vi "Make laser cluster.vi"(0 "445 laser":refnum<visa-resource-name>, 5 "488 laser":refnum<visa-resource-name>, 7 "561 laser":refnum<visa-resource-name>, 9 "640 laser":refnum<visa-resource-name>, 11 "Error In":errorcluster) -> (4 "Laser cluster":T1, 15 "Error Out":errorcluster)   [LabVIEW 2017]
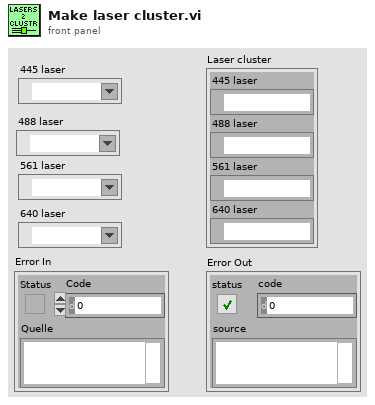
[diagram p1: front panel]
types:
  T1 = cluster{"445 laser":refnum<visa-resource-name>, "488 laser":refnum<visa-resource-name>, "561 laser":refnum<visa-resource-name>, "640 laser":refnum<visa-resource-name>}
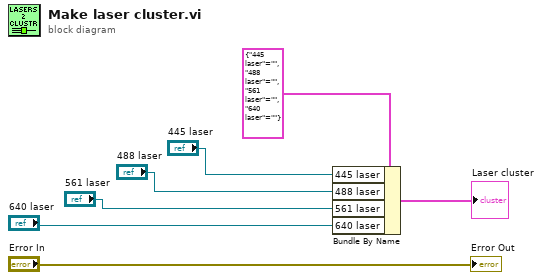
[diagram p0: block diagram]
diagram:
  n1 = Bundle By Name(cluster=T1 {"445 laser"="", "488 laser"="", "561 laser"="", "640 laser"=""} ("input cluster"), "445 laser"="445 laser", "488 laser"="488 laser", "561 laser"="561 laser", "640 laser"="640 laser") -> (→"Laser cluster":T1)
  "Error Out" <- "Error In"
